vi "PRL UTIL Get Control Value.vi"(8 "error in (no error)":errorcluster, 10 "Control Name":string, 11 "VI Reference":refnum<vi>) -> (0 "error out":errorcluster, 3 "Value":variant)   [LabVIEW 2013, in "PMU Recorder Light.lvlib"]
uses:
  PMU Recorder Light.lvlib
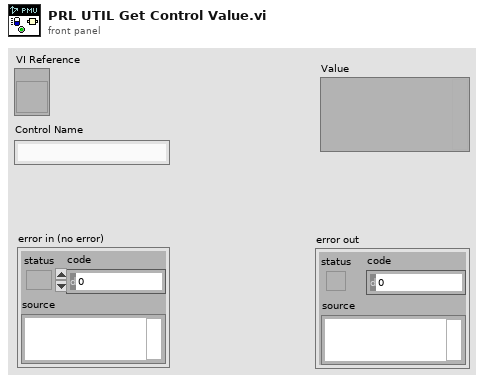
[diagram p1: front panel]
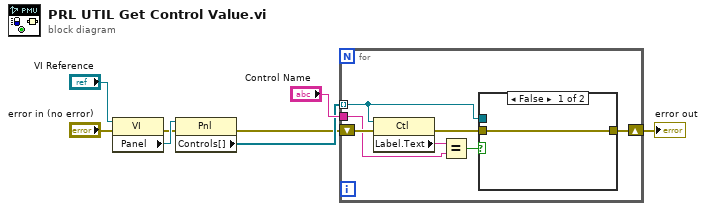
[diagram p0: block diagram]
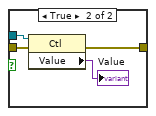
[diagram p2: hidden frame]
diagram:
  n1 = property class="VI"(reference="VI Reference", error in="error in (no error)") -> (error out=w4:errorcluster, "Panel"=w7:refnum<vi>)  [unwired: 1 out]
  n2 = property class="Pnl"(reference=w7, error in=w4) -> (error out=w1:errorcluster, "Controls[]"=w2:refnum<vi>[])  [unwired: 1 out]
  n3 = for {
    tunnel: w2 -> [w13] mode=indexing
    shift-right: [w11] -> w3
    shift-left: w1 -> [w15]
    tunnel: "Control Name" -> [w10]
    n4 = property class="Ctl"(reference=w13, error in=w15) -> (error out=w12:errorcluster, "Label.Text"=w9:string)  [unwired: 1 out]
    n5 = Equal?(x=w9, y=w10) -> (x = y?=w14:bool)
    n6 = case shown="False" w14 {
      tunnel: w13 -> [_ w20]
      tunnel: w12 -> [w16 w18]
      tunnel: [w16 w17] -> w11
      frame False {
      }
      frame True {
        n7 = property class="Ctl"(reference=w20, error in=w18) -> (error out=w17:errorcluster, "Value"=→"Value":variant)  [unwired: 1 out]
      }
    }
  }
  "error out" <- w3
